vi "Get Pack Filed From Logical Screen Descriptor.vi"(8 "error in (no error)":errorcluster caption="错误输入（无错误）", 11 "Gif Image 输入":refnum<class "Gif Image.lvclass"> caption="DNL_LabVIEW Object in") -> (0 "error out":errorcluster caption="错误输出", 3 "Gif Image 输出":refnum<class "Gif Image.lvclass"> caption="DNL_LabVIEW Object out")   [LabVIEW 2012, in "Picture Box Tools.lvlib" / "Gif Image.lvclass"]
uses:
  Gif Image.lvclass
  Control/LSD Packed Field.ctl
  Gif Image.lvclass/Gif Image.ctl
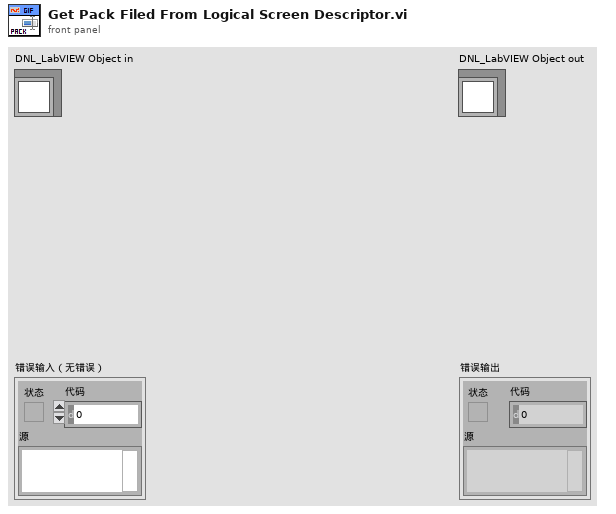
[diagram p1: front panel]
types:
  T1 = typedef "Picture Box Tools.lvlib/Gif Image.lvclass/LSD Packed Field.ctl" = cluster{"Global Color Table Flag":bool, "Color Resolution":u8, "Sort Flag":bool, "Size of Global Color Table":u8}
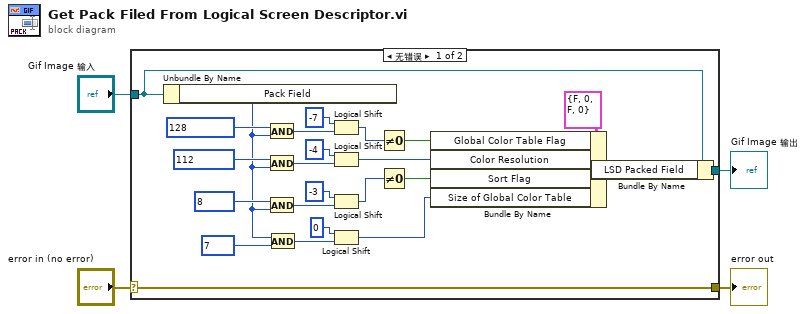
[diagram p0: block diagram]
diagram:
  n1 = case shown="无错误" "error in (no error)" {
    selector: "error in (no error)" -> [w28 w30]
    tunnel: [w28 w30] -> w3
    tunnel: [w5 w29] -> w1
    tunnel: "Gif Image 输入" -> [w7 w29]
    frame No Error {
      n2 = Unbundle By Name(w7) -> ("Pack Field"=w14:u8)
      n3 = And(x=u8 128 ("y"), y=w14) -> (x .and. y?=w25:u8)
      n4 = And(x=u8 112 ("y"), y=w14) -> (x .and. y?=w19:u8)
      n5 = And(x=u8 8 ("y"), y=w14) -> (x .and. y?=w20:u8)
      n6 = And(x=w14, y=u8 7) -> (x .and. y?=w21:u8)
      n7 = Logical Shift(y=-7, x=w25) -> (x << y=w10:u8)
      n8 = Logical Shift(y=-4, x=w19) -> (x << y=w8:u8)
      n9 = Logical Shift(y=-3, x=w20) -> (x << y=w12:u8)
      n10 = Logical Shift(y=0, x=w21) -> (x << y=w13:u8)
      n11 = Not Equal To 0?(x=w10) -> (x != 0?=w9:bool)
      n12 = Not Equal To 0?(x=w12) -> (x != 0?=w11:bool)
      n13 = Bundle By Name(cluster=T1 {"Global Color Table Flag"=FALSE, "Color Resolution"=0, "Sort Flag"=FALSE, "Size of Global Color Table"=0} ("Pack Filed Out"), "Global Color Table Flag"=w9, "Color Resolution"=w8, "Sort Flag"=w11, "Size of Global Color Table"=w13) -> (w6:T1)
      n14 = Bundle By Name(cluster=w7, "LSD Packed Field"=w6) -> (w5:refnum<class "Gif Image.lvclass">)
    }
    frame Error {
    }
  }
  "error out" <- w3
  "Gif Image 输出" <- w1
